vi "Add User Channel Folder_Folder Existing.vi"(8 "error in (no error)":errorcluster, 9 "User Channel Folder Settings":T1, 11 "User Channels Ref":refnum<k24>) -> (0 "error out":errorcluster, 3 "User Channels Ref out":refnum<k24>)   [LabVIEW 2019, in "Simple SysDef API.lvlib"]
uses:
  <userlib>/SimpleSysDef/Simple SysDef API.lvlib
  NationalInstruments.VeriStand.SystemDefinitionAPI
  <userlib>/SimpleSysDef/_SubVIs/Add Folder_Settings.ctl
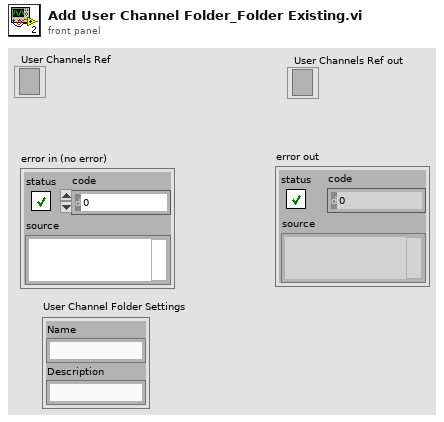
[diagram p1: front panel]
types:
  T1 = typedef "Simple SysDef API.lvlib/Add Folder_Settings.ctl" = cluster{"Name":string, "Description":string}
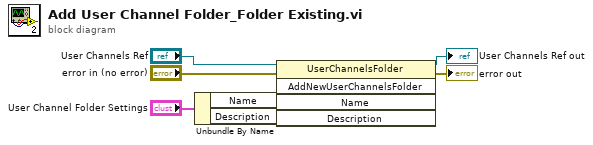
[diagram p0: block diagram]
diagram:
  n1 = Unbundle By Name("User Channel Folder Settings") -> ("Name"=w2:string, "Description"=w1:string)
  n2 = invoke class="UserChannelsFolder" method="AddNewUserChannelsFolder"(reference="User Channels Ref", error in="error in (no error)", "Name"=w2, "Description"=w1) -> (reference out=→"User Channels Ref out":refnum<k24>, error out=→"error out":errorcluster)  [unwired: 1 in, 3 out]
